vi "Simple Read.vi"(4 "Class":refnum<class "Abs_I64 Integer.lvclass">) -> (1 "Value":i64)   [LabVIEW 2021, in "Abs_I64 Integer.lvclass"]
uses:
  Abs_I64 Integer.lvclass
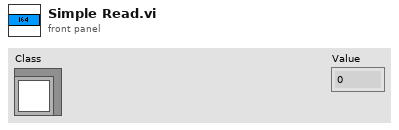
[diagram p1: front panel]
types:
  T1 = typedef "Abs_I64 Integer.lvclass/Type.ctl" = i64
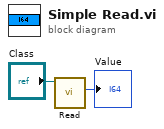
[diagram p0: block diagram]
diagram:
  n1 = call-dynamic "Read.vi"("Double Float.lvclass_340760 in"="Class") -> ("Value"=→"Value":T1)  [unwired: 8 in, 2 out]
